vi "Error_2layerOutX_1layerOutX.vi"(1 "Array_target_ox":dbl[](array[numeric]), 2 "Array_Out_ox":dbl[](array[numeric]), 3 "Array_2layer_Weights_at_Index_hx":dbl[](array[numeric])) -> (0 "Err_outX":dbl)   [LabVIEW 2016]
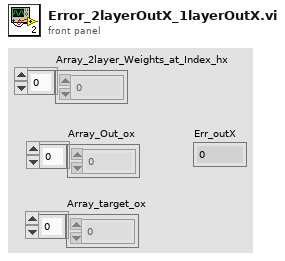
[diagram p1: front panel]
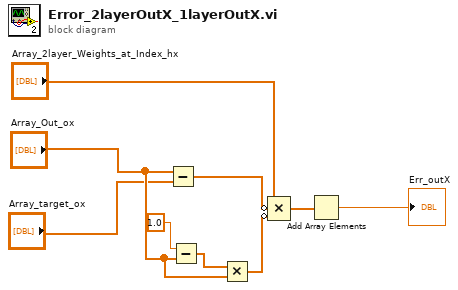
[diagram p0: block diagram]
diagram:
  n1 = Subtract(x="Array_Out_ox", y="Array_target_ox") -> (x-y=w6:dbl[])
  n2 = Subtract(x=1.0, y="Array_Out_ox") -> (x-y=w8:dbl[])
  n3 = Multiply(x=w8, y="Array_Out_ox") -> (x*y=w7:dbl[])
  n4 = Compound Arithmetic op=MULTIPLY("Array_2layer_Weights_at_Index_hx", invert w6, invert w7) -> (w2:dbl[])
  n5 = Add Array Elements(numeric array=w2) -> (sum=→"Err_outX":dbl)
